vi "CtrlGetValue.vi"(0 "reference":refnum<vi>, 1 "error in":errorcluster) -> (2 "variant":variant, 3 "type string":i16[](array[numeric]), 4 "data string":string, 5 "error out":errorcluster)   [LabVIEW 2014]
doc: "Gets the value of a front-panel control.\nParameters:\nany:ctrl, Ctrl.\nErrors:\nNot a Ctrl."
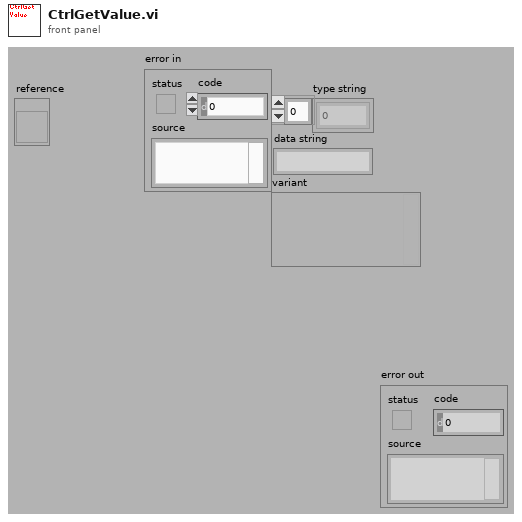
[diagram p1: front panel]
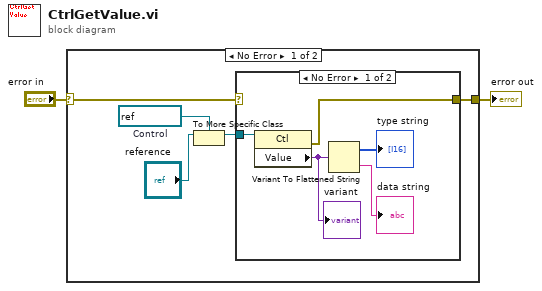
[diagram p0: block diagram]
diagram:
  n1 = case shown="No Error" "error in" {
    selector: "error in" -> [w6 w14]
    tunnel: [w7 w14] -> w2
    frame No Error {
      w4 = refnum<vi> refnum  # Control
      n2 = To More Specific Class(target class=w4, reference="reference") -> (specific class reference=w3:refnum<vi>)  [unwired: 1 in, 1 out]
      n3 = case shown="No Error" w6 {
        selector: w6 -> [_ w13]
        tunnel: [w12 w13] -> w7
        tunnel: w3 -> [w11 _]
        frame No Error {
          n4 = property class="Ctl"(reference=w11) -> (error out=w12:errorcluster, "Value"=w8:variant)  [unwired: 1 in, 1 out]
          "variant" <- w8
          n5 = Variant To Flattened String(Variant=w8) -> (data string=→"data string":string, 1:→"type string":i16[])
        }
        frame Error {
        }
      }
    }
    frame Error {
    }
  }
  "error out" <- w2
